vi "Render Text Blended.vi"(9 "Colour":u32(colorbox), 10 "Text":string, 11 "Font Pointer":u32 format="%.0x") -> (3 "Surface Pointer":u32 format="%.0x")   [LabVIEW 2015, in "LibSDL2_TTF.lvlib"]
uses:
  LibSDL2_TTF.lvlib
  LibSDL2 Wrapper/DLL/SDL2_ttf.dll
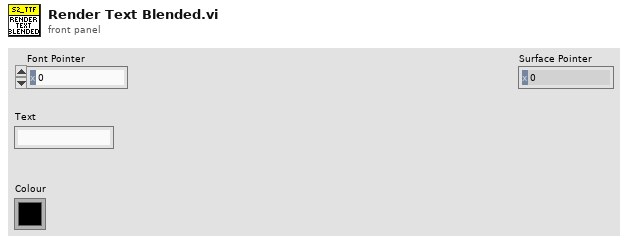
[diagram p1: front panel]
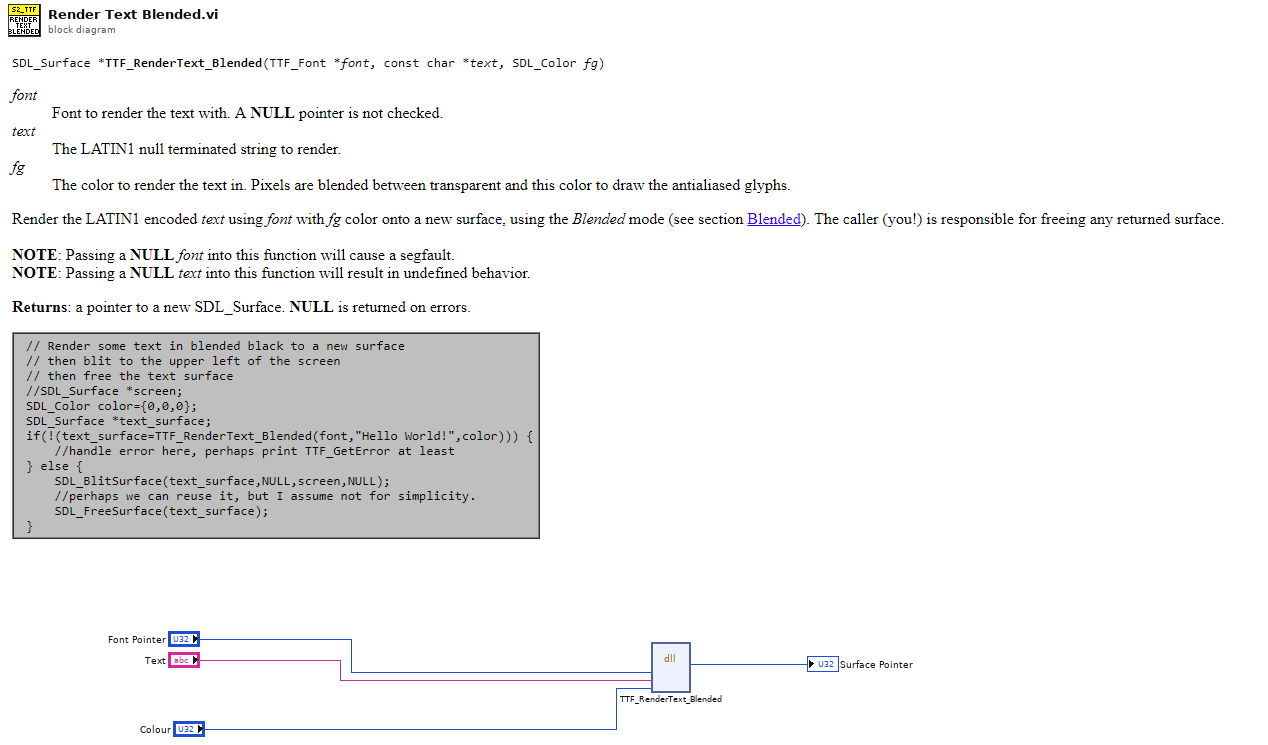
[diagram p0: block diagram]
diagram:
  n1 = dll-call lib="C:/dev/PGS/LabSDL2/Source/Libraries/LibSDL2 Wrapper/DLL/SDL2_ttf.dll" fn="TTF_RenderText_Blended"("Font Pointer"="Font Pointer", "Text"="Text", "Colour"="Colour") -> ("Surface Pointer"=→"Surface Pointer":u32)  [unwired: 6 in, 2 out]
